vi "Get MDIFBlock Info.vi"(8 "error in (no error)":errorcluster, 11 "MDIF Block Refnum in":refnum<k24>) -> (0 "error out":errorcluster, 3 "MDIF Block":T1)   [LabVIEW 2023, in "NI_HFNetworkAnalysis.lvlib"]
uses:
  NI_HFNetworkAnalysis.lvlib
  Controls/MDIF Block.ctl
  C:/srd-semi-rfcal-software/AuxTools/STSRFFixtureCharactUtility/Source/Code Modules/Fixture/Dependencies/HFNetworkAnalysis/Support Files/NACE.Utils.Data.dll
  Support Files/NACE.Utils.Data.dll
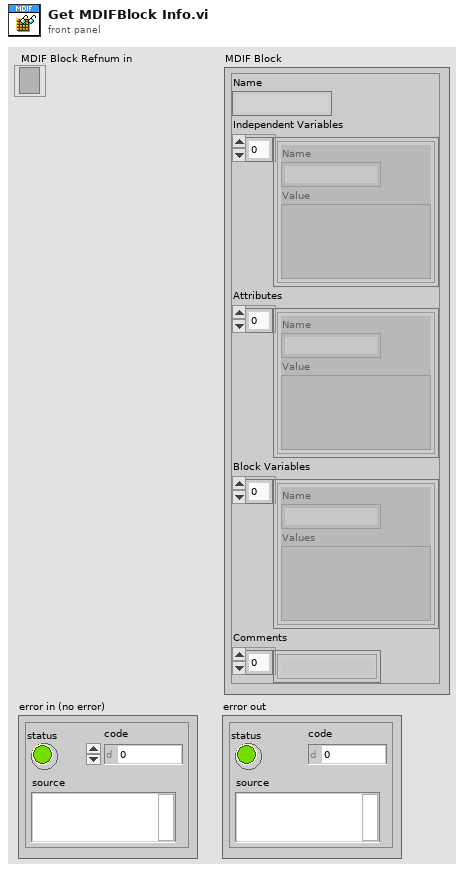
[diagram p1: front panel]
types:
  T1 = typedef "NI_HFNetworkAnalysis.lvlib/MDIF Block.ctl" = cluster{"Name":string, "Independent Variables":cluster{"Name":string, "Value":variant}[], "Attributes":cluster{"Name":string, "Value":variant}[], "Block Variables":cluster{"Name":string, "Values":variant}[], "Comments":string[]}
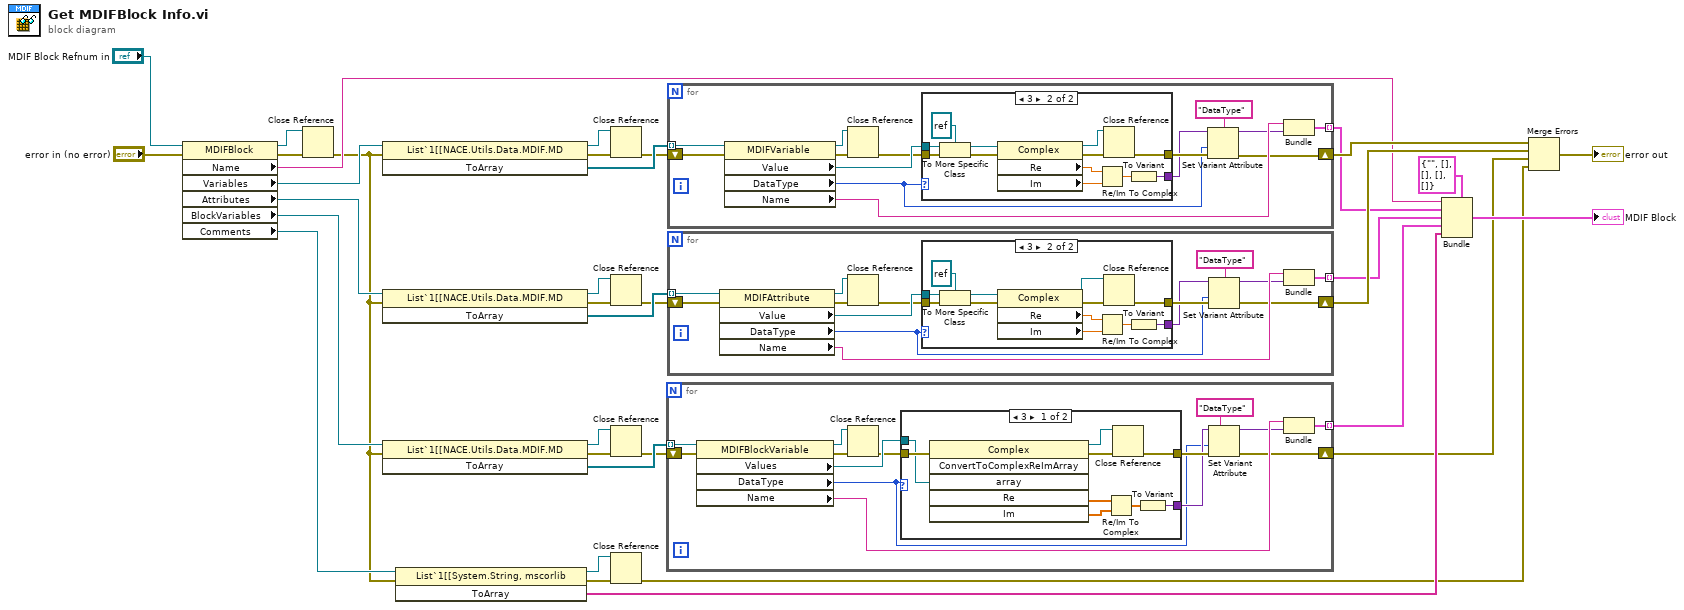
[diagram p0: block diagram]
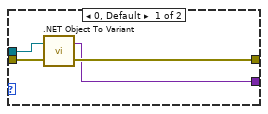
[diagram p2: hidden frame]
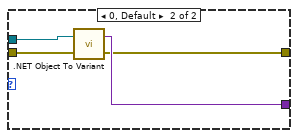
[diagram p3: hidden frame]
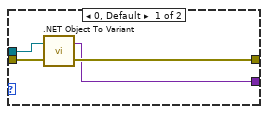
[diagram p4: hidden frame]
diagram:
  n1 = property class="MDIFBlock"(reference="MDIF Block Refnum in", error in="error in (no error)") -> (reference out=w10:refnum<k24>, error out=w12:errorcluster, "Name"=w21:string, "Variables"=w19:refnum<k24>, "Attributes"=w25:refnum<k24>, "BlockVariables"=w28:refnum<k24>, "Comments"=w29:refnum<k24>)
  n2 = Close Reference(reference=w10, error in (no error)=w12) -> (error out=w11:errorcluster)
  n3 = invoke class="List`1[[NACE.Utils.Data.MDIF.MD" method="ToArray"(reference=w19, error in=w11) -> (reference out=w8:refnum<k24>, error out=w20:errorcluster, "ToArray"=w16:refnum<k24>[])  [unwired: 1 in]
  n4 = invoke class="List`1[[NACE.Utils.Data.MDIF.MD" method="ToArray"(reference=w25, error in=w11) -> (reference out=w6:refnum<k24>, error out=w24:errorcluster, "ToArray"=w15:refnum<k24>[])  [unwired: 1 in]
  n5 = invoke class="List`1[[NACE.Utils.Data.MDIF.MD" method="ToArray"(reference=w28, error in=w11) -> (reference out=w4:refnum<k24>, error out=w23:errorcluster, "ToArray"=w14:refnum<k24>[])  [unwired: 1 in]
  n6 = invoke class="List`1[[System.String, mscorlib" method="ToArray"(reference=w29, error in=w11) -> (reference out=w2:refnum<k24>, error out=w30:errorcluster, "ToArray"=w13:string[])  [unwired: 1 in]
  n7 = Close Reference(reference=w8, error in (no error)=w20) -> (error out=w9:errorcluster)
  n8 = Close Reference(reference=w6, error in (no error)=w24) -> (error out=w7:errorcluster)
  n9 = Close Reference(reference=w4, error in (no error)=w23) -> (error out=w5:errorcluster)
  n10 = Close Reference(reference=w2, error in (no error)=w30) -> (error out=w3:errorcluster)
  n11 = for {
    tunnel: w14 -> [w47] mode=indexing
    tunnel: [w48] -> w27 mode=indexing
    shift-right: [w40] -> w1
    shift-left: w5 -> [w49]
    n12 = property class="MDIFBlockVariable"(reference=w47, error in=w49) -> (reference out=w42:refnum<k24>, error out=w44:errorcluster, "Values"=w45:refnum<k24>, "DataType"=w36:i32, "Name"=w46:string)
    n13 = Close Reference(reference=w42, error in (no error)=w44) -> (error out=w43:errorcluster)
    n14 = case shown="3" w36 {
      tunnel: w45 -> [w57 w61]
      tunnel: w43 -> [w58 w62]
      tunnel: [w51 w59] -> w41
      tunnel: [w56 w60] -> w39
      frame 3 {
        n15 = invoke class="Complex" method="ConvertToComplexReImArray"(error in=w58, "array"=w57) -> (reference out=w50:refnum<k24>, error out=w55:errorcluster, "Re"=w54:dbl[], "Im"=w53:dbl[])  [unwired: 4 in, 2 out]
        n16 = Re/Im To Complex(1:w53, 2:w54) -> (0:w52:cdb[])
        n17 = Close Reference(reference=w50, error in (no error)=w55) -> (error out=w51:errorcluster)
        n18 = To Variant(anything=w52) -> (Variant=w56:variant)
      }
      frame 0, Default {
        n19 = call <vilib>:".NET Object To Variant.vi"("error in (no error)"=w62, ".NET object"=w61) -> ("error out"=w59:errorcluster, "variant"=w60:variant)
      }
    }
    n20 = Set Variant Attribute(Variant=w39, name="DataType", value=w36, error in=w41) -> (Variant out=w38:variant, error out=w40:errorcluster)  [unwired: 1 out]
    n21 = Bundle("Name"=w46, "variant"=w38) -> (w48:cluster{"Name":string, "variant":variant})  [unwired: 1 in]
  }
  n22 = for {
    tunnel: w16 -> [w72] mode=indexing
    tunnel: [w73] -> w22 mode=indexing
    shift-right: [w67] -> w33
    shift-left: w9 -> [w71]
    n23 = property class="MDIFVariable"(reference=w72, error in=w71) -> (reference out=w69:refnum<k24>, error out=w76:errorcluster, "Value"=w75:refnum<k24>, "DataType"=w63:i32, "Name"=w74:string)
    n24 = Close Reference(reference=w69, error in (no error)=w76) -> (error out=w70:errorcluster)
    n25 = case shown="3" w63 {
      tunnel: w75 -> [w80 w92]
      tunnel: w70 -> [w79 w86]
      tunnel: [w77 w84] -> w65
      tunnel: [w78 w82] -> w68
      frame 0, Default {
        n26 = call <vilib>:".NET Object To Variant.vi"("error in (no error)"=w79, ".NET object"=w80) -> ("error out"=w78:errorcluster, "variant"=w77:variant)
      }
      frame 3 {
        n27 = To More Specific Class(target class=refnum<k24> refnum, reference=w92, error in=w86) -> (specific class reference=w89:refnum<k24>, error out=w90:errorcluster)
        n28 = property class="Complex"(reference=w89, error in=w90) -> (reference out=w81:refnum<k24>, error out=w83:errorcluster, "Re"=w87:dbl, "Im"=w88:dbl)
        n29 = Re/Im To Complex(1:w88, 2:w87) -> (0:w85:cdb)
        n30 = Close Reference(reference=w81, error in (no error)=w83) -> (error out=w82:errorcluster)
        n31 = To Variant(anything=w85) -> (Variant=w84:variant)
      }
    }
    n32 = Set Variant Attribute(Variant=w65, name="DataType", value=w63, error in=w68) -> (Variant out=w64:variant, error out=w67:errorcluster)  [unwired: 1 out]
    n33 = Bundle("Name"=w74, "Variant"=w64) -> (w73:cluster{"Name":string, "Variant":variant})  [unwired: 1 in]
  }
  n34 = for {
    tunnel: w15 -> [w104] mode=indexing
    tunnel: [w102] -> w26 mode=indexing
    shift-right: [w99] -> w34
    shift-left: w7 -> [w105]
    n35 = property class="MDIFAttribute"(reference=w104, error in=w105) -> (reference out=w97:refnum<k24>, error out=w100:errorcluster, "Value"=w101:refnum<k24>, "DataType"=w93:i32, "Name"=w103:string)
    n36 = Close Reference(reference=w97, error in (no error)=w100) -> (error out=w98:errorcluster)
    n37 = case shown="3" w93 {
      tunnel: w101 -> [w109 w121]
      tunnel: w98 -> [w108 w115]
      tunnel: [w106 w113] -> w95
      tunnel: [w107 w111] -> w99
      frame 0, Default {
        n38 = call <vilib>:".NET Object To Variant.vi"("error in (no error)"=w108, ".NET object"=w109) -> ("error out"=w107:errorcluster, "variant"=w106:variant)
      }
      frame 3 {
        n39 = To More Specific Class(target class=refnum<k24> refnum, reference=w121, error in=w115) -> (specific class reference=w118:refnum<k24>, error out=w119:errorcluster)
        n40 = property class="Complex"(reference=w118, error in=w119) -> (reference out=w110:refnum<k24>, error out=w112:errorcluster, "Re"=w116:dbl, "Im"=w117:dbl)
        n41 = Re/Im To Complex(1:w117, 2:w116) -> (0:w114:cdb)
        n42 = Close Reference(reference=w110, error in (no error)=w112) -> (error out=w111:errorcluster)
        n43 = To Variant(anything=w114) -> (Variant=w113:variant)
      }
    }
    n44 = Set Variant Attribute(Variant=w95, name="DataType", value=w93) -> (Variant out=w94:variant)  [unwired: 1 in, 2 out]
    n45 = Bundle("Name"=w103, "Variant"=w94) -> (w102:cluster{"Name":string, "Variant":variant})  [unwired: 1 in]
  }
  n46 = Bundle(cluster=T1 {"Name"="", "Independent Variables"=[], "Attributes"=[], "Block Variables"=[], "Comments"=[]} ("MDIF Block"), "Name"=w21, "Independent Variables"=w22, "Attributes"=w26, "Block Variables"=w27, "Comments"=w13) -> (→"MDIF Block":T1)
  n47 = Merge Errors(w33, w34, w1, w3) -> (→"error out":errorcluster)
